vi "ExtCall.vi"(8 "error in (no error)":errorcluster, 9 "Val":variant, 10 "Tag":u16, 11 "Square in":refnum<class "Rigol DG822 Square.lvclass">) -> (0 "error out":errorcluster, 1 "Response":variant, 3 "Square out":refnum<class "Rigol DG822 Square.lvclass">)   [LabVIEW 2021, in "Rigol DG822 UI.lvlib" / "Rigol DG822 Square.lvlib" / "Rigol DG822 Square.lvclass"]
uses:
  Rigol DG822 Square.lvclass
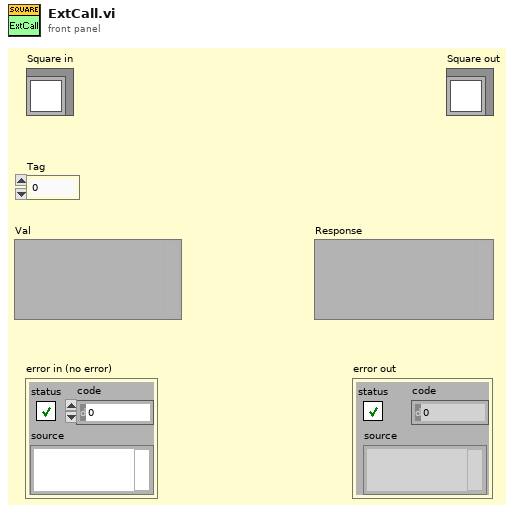
[diagram p1: front panel]
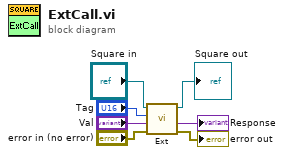
[diagram p0: block diagram]
diagram:
  n1 = call "Ext.vi"("error in (no error)"="error in (no error)", "Val"="Val", "Tag"="Tag", "Square in"="Square in") -> ("error out"=→"error out":errorcluster, "Parsed"=→"Response":variant, "Square out"=→"Square out":refnum<class "Rigol DG822 Square.lvclass">)  [unwired: 5 in]
